vi "Fake Service Location FGV.vi"(8 "error in":errorcluster, 9 "unique id in":u64, 10 "resolve service request":T1, 11 "action":T3) -> (0 "error out":errorcluster, 1 "unique id out":u64, 3 "service location":T2)   [LabVIEW 2020, in "MeasurementServerTests.lvlib" / "Discovery Tests.lvlib"]
uses:
  Discovery Tests.lvlib
  Runtime/MeasurementLink Discovery V1/MeasurementLink Discovery V1.lvlib
  Fake Resolve Service.vi
  Runtime/MeasurementLink Discovery V1/TypeDefs/Service Location FGV Action.ctl
  Runtime/MeasurementLink Discovery Client/RPC Messages/ni_measurementlink_discovery_v1_ServiceLocation.ctl
  Runtime/MeasurementLink Discovery Client/MeasurementLink Discovery Client.lvlib
  Runtime/MeasurementLink Discovery Client/RPC Messages/ni_measurementlink_discovery_v1_ResolveServiceRequest.ctl
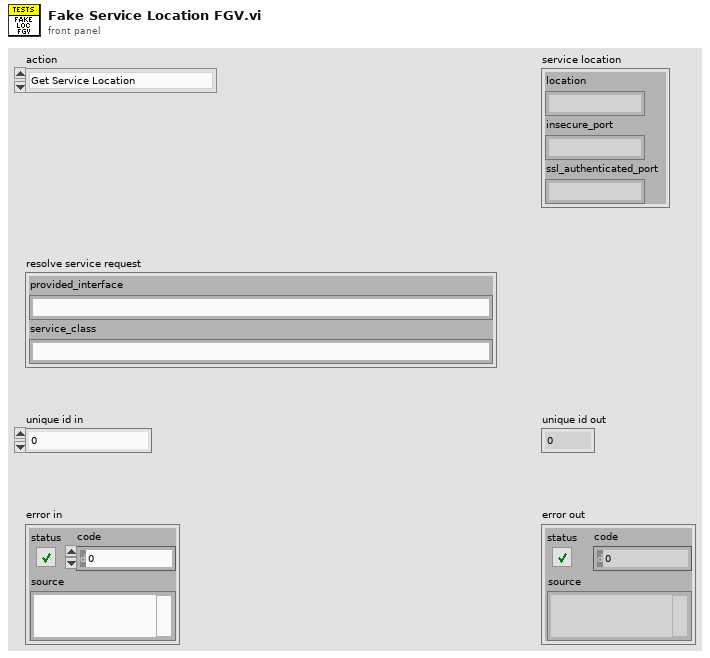
[diagram p1: front panel]
types:
  T1 = typedef "MeasurementLink Discovery Client.lvlib/ni_measurementlink_discovery_v1_ResolveServiceRequest.ctl" = cluster{"provided_interface":string, "service_class":string}
  T2 = typedef "MeasurementLink Discovery Client.lvlib/ni_measurementlink_discovery_v1_ServiceLocation.ctl" = cluster{"location":string, "insecure_port":string, "ssl_authenticated_port":string}
  T3 = typedef "MeasurementLink Discovery V1.lvlib/Service Location FGV Action.ctl" = enum16{"Get Service Location", "Reresolve Service Location"}
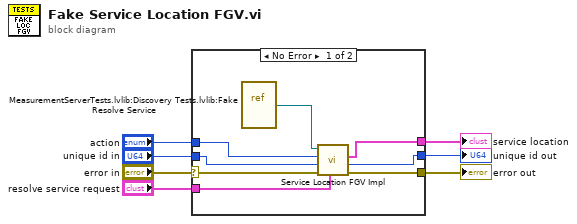
[diagram p0: block diagram]
diagram:
  n1 = case shown="No Error" "error in" {
    selector: "error in" -> [w15 w16]
    tunnel: [w13 w16] -> w7
    tunnel: "unique id in" -> [w14 _]
    tunnel: [w12 _] -> w1
    tunnel: "action" -> [w11 _]
    tunnel: [w10 _] -> w3
    tunnel: "resolve service request" -> [w9 _]
    frame No Error {
      n2 = vi-ref "MeasurementServerTests.lvlib:Discovery Tests.lvlib:Fake Resolve Service.vi"() -> (w8:refnum<vi>)
      n3 = call "Service Location FGV Impl.vi"("resolve service request"=w9, "error in"=w15, "location unique id in"=w14, "action"=w11, "resolve vi reference"=w8) -> ("error out"=w13:errorcluster, "location unique id out"=w12:u64, "service location"=w10:T2)  [unwired: 4 in]
    }
    frame Error {
    }
  }
  "error out" <- w7
  "service location" <- w3
  "unique id out" <- w1
